vi "Set Ready to Close.vi"(8 "error in (no error)":errorcluster, 11 "navX - Interface in":refnum<class "navX - Interface.lvclass">) -> (0 "error out":errorcluster, 3 "navX - Interface out":refnum<class "navX - Interface.lvclass">)   [LabVIEW 2015, in "navX Library v3.lvlib" / "navX - Interface.lvclass"]
uses:
  navX - Interface.lvclass
  navX - Interface.lvclass/navX - Interface.ctl
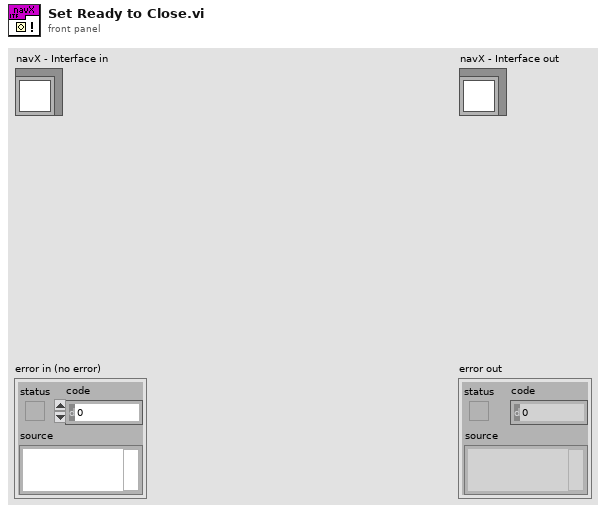
[diagram p1: front panel]
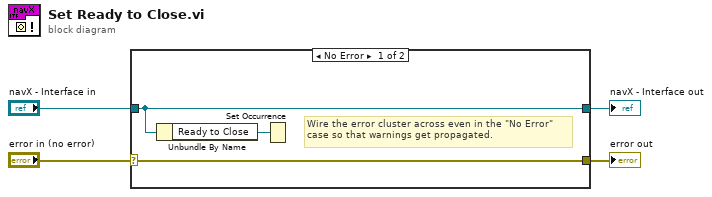
[diagram p0: block diagram]
diagram:
  n1 = case shown="No Error" "error in (no error)" {
    selector: "error in (no error)" -> [w7 w9]
    tunnel: [w7 w9] -> w3
    tunnel: [w6 w8] -> w1
    tunnel: "navX - Interface in" -> [w6 w8]
    frame No Error {
      # "Wire the error cluster across even in the \"No Error\"\ncase so that warnings get propagated."
      n2 = Unbundle By Name(w6) -> ("Ready to Close"=w5:refnum<k4>)
      n3 = Set Occurrence(w5) -> ()
    }
    frame Error {
    }
  }
  "error out" <- w3
  "navX - Interface out" <- w1
